vi "Read Tsp.vi"(8 "error in (no error)":errorcluster, 11 "mTEC Data in":refnum<class "mTEC Data.lvclass">) -> (0 "error out":errorcluster, 2 "Tsp":dbl, 3 "mTEC Data out":refnum<class "mTEC Data.lvclass">)   [LabVIEW 2014, in "Meerstetter Lib.lvlib" / "mTEC Data.lvclass"]
uses:
  mTEC Data.lvclass
  mTEC Data.lvclass/mTEC Data.ctl
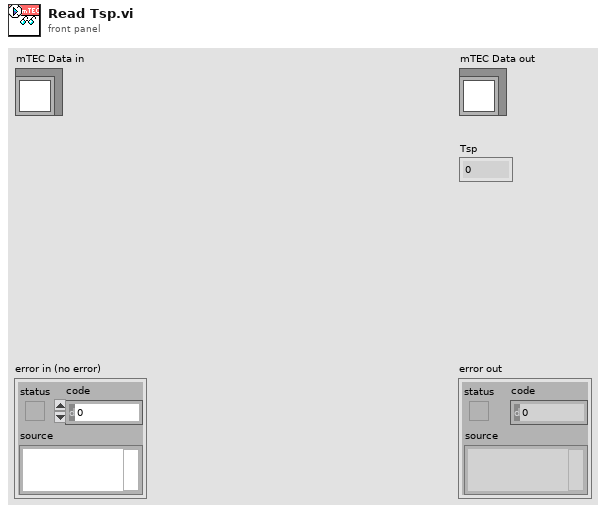
[diagram p1: front panel]
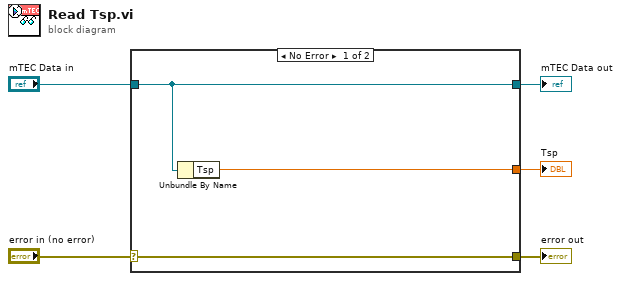
[diagram p0: block diagram]
diagram:
  n1 = case shown="No Error" "error in (no error)" {
    selector: "error in (no error)" -> [w8 w9]
    tunnel: [w8 w9] -> w4
    tunnel: [w7 w10] -> w2
    tunnel: "mTEC Data in" -> [w7 w10]
    tunnel: [w6 _] -> w1
    frame No Error {
      n2 = Unbundle By Name(w7) -> ("Tsp"=w6:dbl)
    }
    frame Error {
    }
  }
  "error out" <- w4
  "mTEC Data out" <- w2
  "Tsp" <- w1
